vi "Start.vi"(8 "error in (no error)":errorcluster, 10 "Message in":refnum<class "StartMessage.lvclass">, 11 "ImageStack in":refnum<class "ImageStack.lvclass">) -> (0 "error out":errorcluster, 3 "ImageStack out":refnum<class "ImageStack.lvclass">)   [LabVIEW 2012, in "ImageStack.lvclass"]
doc: "This member function is called when the statemachine in the run.vi receives an 'start' command. It relays the message to all observers of the component.\n\nOverride this member function in your derived class if you need additional start functionality (but don't forget to call the parent method)."
uses:
  ImageStack.lvclass
  <vilib>/Distrio/Murmex/Murmex/Murmex.lvclass
  <vilib>/Distrio/Murmex/StartMessage/StartMessage.lvclass
  <vilib>/Distrio/Murmex/StartMessage/run mode enum.ctl
panel:
  # "This member function is called when the statemachine in the run.vi receives an 'start' command. It relays the message to all observers of the component.\n\nOverride this member function in your derived class if you need additional start functionality (but don't forget to call the parent method)."
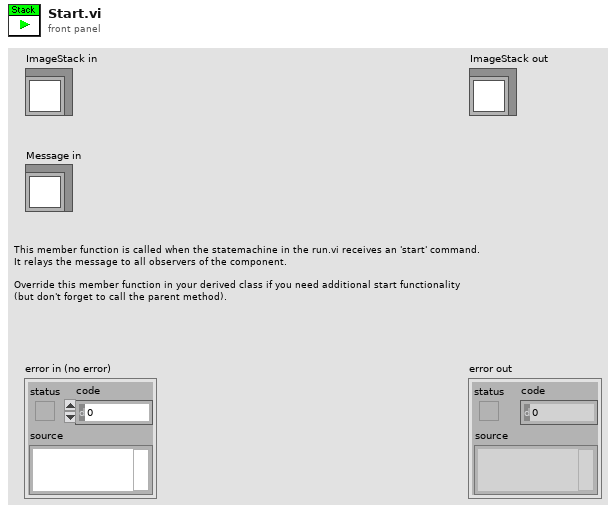
[diagram p1: front panel]
types:
  T1 = typedef "Murmex.lvlib/StartMessage.lvclass/run mode enum.ctl" = enum16{"infinite", "finite"}
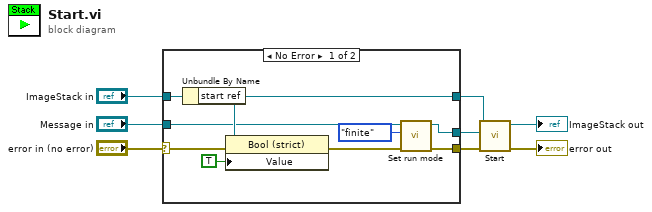
[diagram p0: block diagram]
diagram:
  n1 = case shown="No Error" "error in (no error)" {
    selector: "error in (no error)" -> [w16 w18]
    tunnel: "ImageStack in" -> [w9 w20]
    tunnel: "Message in" -> [w13 w19]
    tunnel: [w11 w19] -> w5
    tunnel: [w10 w18] -> w4
    tunnel: [w9 w20] -> w3
    frame No Error {
      n2 = Unbundle By Name(w9) -> ("start ref"=w17:refnum<vi>)
      n3 = property class="Bool (strict)"(reference=w17, error in=w16, "Value"=TRUE) -> (error out=w14:errorcluster)  [unwired: 1 out]
      n4 = call <vilib>:"Set run mode.vi"("error in (no error)"=w14, "run mode"=run_mode_enum."finite", "StartMessage in"=w13) -> ("error out"=w10:errorcluster, "StartMessage out"=w11:refnum<class "StartMessage.lvclass">)  [unwired: 7 in]
    }
    frame Error {
    }
  }
  n5 = call-parent "Start.vi"("error in (no error)"=w4, "Message in"=w5, "Murmex in"=w3) -> ("error out"=→"error out":errorcluster, "Murmex out"=→"ImageStack out":refnum<class "ImageStack.lvclass">)  [unwired: 7 in]
